vi "c ctre phoenixpro get configs no malloc.vi"(0 "context":u32(ring) items=["ContextAPI", "ContextDiagServer"], 1 "str":string, 2 "useDid":bool, 5 "network":string, 7 "deviceHash":i32, 9 "timeoutSeconds":dbl, 11 "error in (no error)":errorcluster, 12 "str_len":u32) -> (3 "str out":string, 4 "function return":i32, 15 "error out":errorcluster)   [LabVIEW 2020, in "CTRE_PhoenixTools.lvlib"]
doc: "CTREXPORT int c_ctre_phoenixpro_get_configs_no_malloc(\n Context context,\n const char *network,\n int deviceHash,\n double timeoutSeconds,\n char *str,\n uint32_t str_len,\n bool useDid);"
uses:
  CTRE_PhoenixTools.lvlib
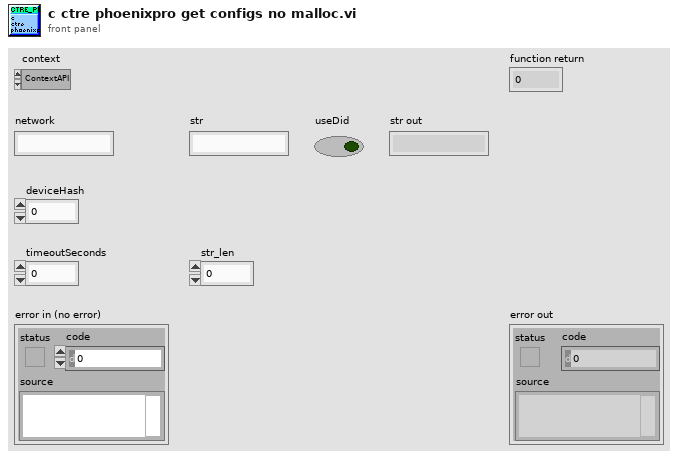
[diagram p1: front panel]
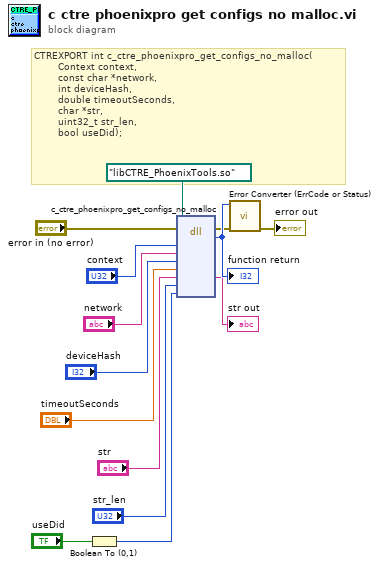
[diagram p0: block diagram]
diagram:
  # "CTREXPORT int c_ctre_phoenixpro_get_configs_no_malloc(\n        Context context,\n        const char *network,\n        int deviceHash,\n        double timeoutSeconds,\n        char *str,\n        uint32_t str_len,\n        bool useDid);"
  n1 = Boolean To (0,1)(Boolean="useDid") -> (0, 1=w5:i16)
  n2 = dll-call lib="?" fn="c_ctre_phoenixpro_get_configs_no_malloc"(path in=path "libCTRE_PhoenixTools.so", error in="error in (no error)", "context"="context", "network"="network", "deviceHash"="deviceHash", "timeoutSeconds"="timeoutSeconds", "str"="str", "str_len"="str_len", "useDid"=w5) -> (error out=w3:errorcluster, w14:i32, "str"=→"str out":string)  [unwired: 7 in, 1 out]
  "function return" <- w14
  n3 = call "Error Converter (ErrCode or Status).vi"("error in (no error)"=w3, "error code"=w14) -> ("error out"=→"error out":errorcluster)  [unwired: 9 in]
